vi "Move Panel to Origin.vi"(0 "VI Reference":refnum<vi>) -> ()   [LabVIEW 2020, in "Utilities.lvlib"]
doc: "Moves the pane to the origin. This helps when designing a front panel since you can make the assumption that the pane's origin will be placed at the top-left of the window if this VI is called."
uses:
  Utilities.lvlib
  <vilib>/Utility/miscctls.llb/LVPointTypeDef.ctl
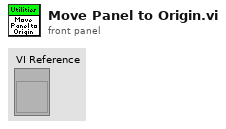
[diagram p1: front panel]
types:
  T1 = typedef "LVPointTypeDef.ctl" = cluster{"Horizontal":i16, "Vertical":i16}
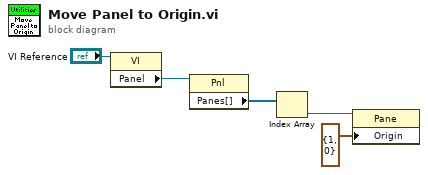
[diagram p0: block diagram]
diagram:
  n1 = property class="VI"(reference="VI Reference") -> ("Panel"=w5:refnum<vi>)  [unwired: 1 in, 2 out]
  n2 = property class="Pnl"(reference=w5) -> ("Panes[]"=w4:refnum<vi>[])  [unwired: 1 in, 2 out]
  n3 = Index Array(array=w4) -> (element=w3:refnum<vi>)  [unwired: 1 in]
  n4 = property class="Pane"(reference=w3, "Origin"=T1 {"Horizontal"=1, "Vertical"=0}) -> ()  [unwired: 1 in, 2 out]
